vi "ABR-Init Raw Data File.vi"(0 "Runtime in":T1, 11 "error in (no error)":errorcluster) -> (4 "Runtime out":T1, 8 "refnum out":refnum<file>, 15 "error out":errorcluster)   [LabVIEW 2020]
uses:
  Typedefs/ABR-Runtime Data.ctl
  epl-vi-lib/Signal Synthesis VIs/4th Generation/Classes/SignalManager/SignalManager.lvclass
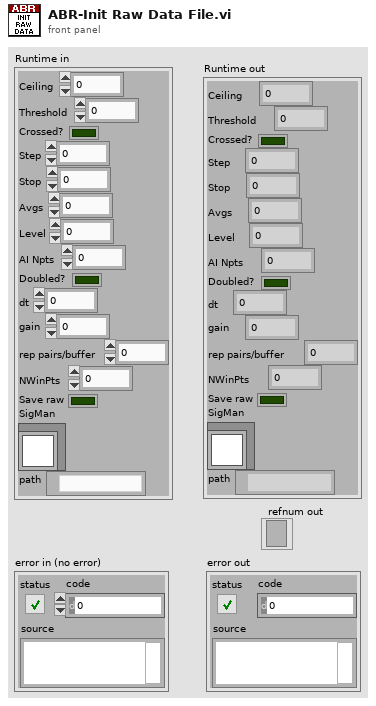
[diagram p1: front panel]
types:
  T1 = typedef "ABR-Runtime Data.ctl" = cluster{"Ceiling":dbl, "Threshold":dbl, "Crossed?":bool, "Step":dbl, "Stop":i32, "Avgs":i32, "Level":dbl, "AI Npts":i32, "Doubled?":bool, "dt":dbl, "gain":dbl, "rep pairs/buffer":i32, "NWinPts":i32, "Save raw":bool, "SigMan":refnum<class "SignalManager.lvclass">, "path":path}
  T2 = enum16{"open", "replace", "create", "open or create", "replace or create", "replace or create with confirmation"}
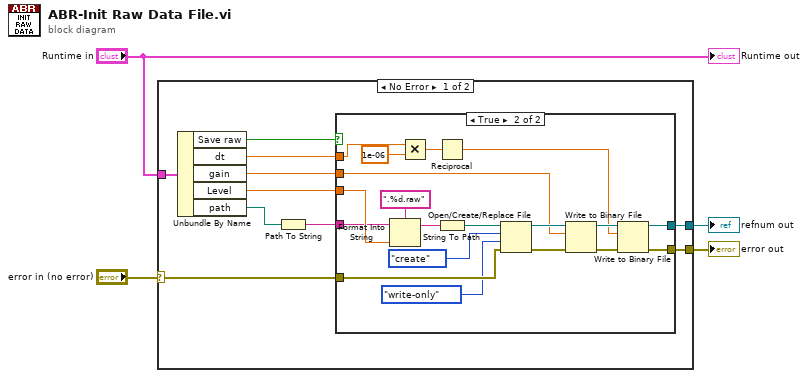
[diagram p0: block diagram]
diagram:
  n1 = case shown="No Error" "error in (no error)" {
    selector: "error in (no error)" -> [w8 w35]
    tunnel: "Runtime in" -> [w12 _]
    tunnel: [w10 _] -> w3
    tunnel: [w7 w35] -> w1
    frame No Error {
      n2 = Unbundle By Name(w12) -> ("Save raw"=w9:bool, "dt"=w6:dbl, "gain"=w11:dbl, "Level"=w14:dbl, "path"=w5:path)
      n3 = Path To String(path=w5) -> (string=w13:string)
      n4 = case shown="True" w9 {
        tunnel: w14 -> [_ w33]
        tunnel: w13 -> [_ w30]
        tunnel: w11 -> [_ w27]
        tunnel: [_ w20] -> w10
        tunnel: w8 -> [w15 w26]
        tunnel: [w15 w22] -> w7
        tunnel: w6 -> [_ w19]
        frame False {
        }
        frame True {
          n5 = Format Into String(format string=".%d.raw", initial string=w30, w33) -> (resulting string=w32:string)  [unwired: 1 in, 1 out]
          n6 = Multiply(x=w19, y=1e-06) -> (x*y=w17:dbl)
          n7 = Reciprocal(x=w17) -> (1/x=w16:dbl)
          n8 = String To Path(string=w32) -> (path=w31:path)
          n9 = Open/Create/Replace File(file path (use dialog)=w31, error in=w26, operation (0:open)=T2."create", access (0:read/write)=enum16{"read/write", "read-only", "write-only"}."write-only") -> (refnum out=w28:refnum<file>, error out=w29:errorcluster)  [unwired: 2 in, 1 out]
          n10 = Write to Binary File(file (use dialog)=w28, data=w27, error in=w29) -> (refnum out=w21:refnum<file>, error out=w23:errorcluster)  [unwired: 3 in, 1 out]
          n11 = Write to Binary File(file (use dialog)=w21, data=w16, error in=w23) -> (refnum out=w20:refnum<file>, error out=w22:errorcluster)  [unwired: 3 in, 1 out]
        }
      }
    }
    frame Error {
    }
  }
  "error out" <- w1
  "refnum out" <- w3
  "Runtime out" <- "Runtime in"
